vi "Save dat File (Core).vi"(0 "File path in":path, 5 "Attributes":string[][](array[string]), 7 "Channels names":string[](array[string]), 9 "Data":sgl[][](array[numeric]) format="%.2p", 11 "error in":errorcluster, 12 "Cut Data at first NaN":bool=TRUE caption="Cut Data at first NaN? (T)") -> (4 "File path out":path, 15 "error out":errorcluster)   [LabVIEW 2017, in "Nanonis Prog Interface.lvlib"]
doc: "<b>Saves a .dat file.</b>\n\nIt saves the attributes in the header, and then the channels names and the corresponding data into a .dat file.\n\nThis function is the core of the Save dat File function, and it's not password-protected so that the user has access to the code.\n\nIf file dialog and/or automated file naming are needed, the user should use the Save dat File function instead.\n\n<B>File path in</B>: full path input of the saved file.\n<B>Attributes</B>: the first column should be fill in with the attribute name, and the second column with the attribute value.\n<B>Channels names</B>: these are set as column headers in the file. The signals names are available in Signals palette through Signal Names Get function.\n<B>Data</B>: saved data in 2D array format. Each row represents one channel.\n<B>Cut Data at first NaN</B>: optional input to avoid saving Not a Number values into the file. It is set to True by default.\n\n<B>File path out</B>: full path output of the saved fle.\n\n- Nanonis Programming Interface -"
uses:
  Nanonis Prog Interface.lvlib
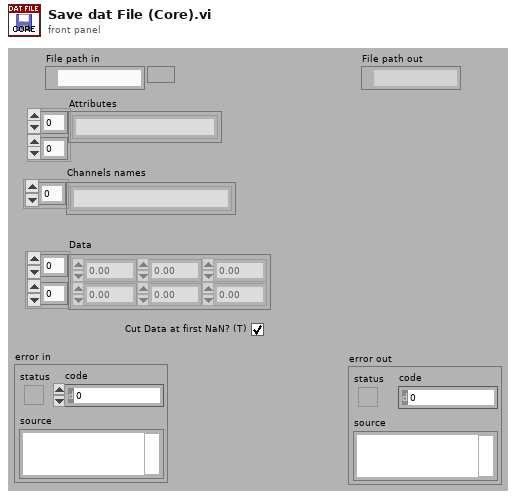
[diagram p1: front panel]
types:
  T1 = enum16{"open", "replace", "create", "open or create", "replace or create", "replace or create with confirmation"}
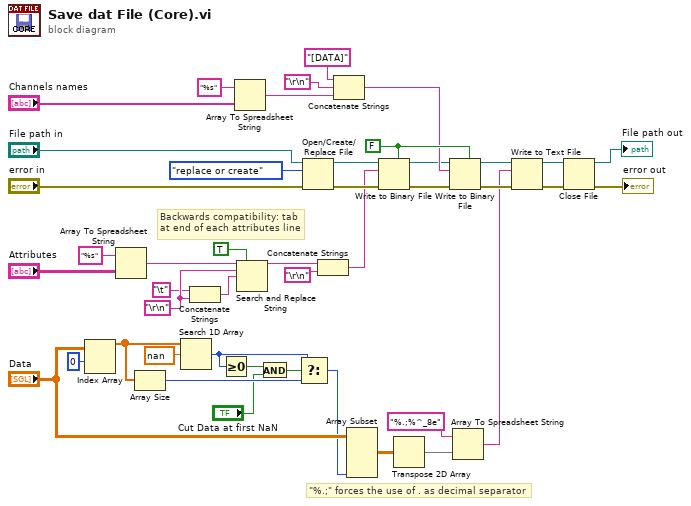
[diagram p0: block diagram]
diagram:
  w4 = "\r\n"
  w33 = FALSE ("prepend array or string size? (T)")
  # "Backwards compatibility: tab at end of each attributes line"
  # "\"%.;\" forces the use of . as decimal separator"
  n1 = Index Array(array="Data", index (row)=0 ("disabled index (col)")) -> (element=w16:sgl[])  [unwired: 1 in]
  n2 = Array To Spreadsheet String(array="Attributes", 3:"%s" ("format string")) -> (spreadsheet string=w6:string)  [unwired: 1 in]
  n3 = Array Size(array=w16) -> (size(s)=w23:i32)
  n4 = Search 1D Array(1D array=w16, element=sgl nan) -> (index of element=w17:i32)  [unwired: 1 in]
  n5 = Concatenate Strings("\t", w4) -> (w2:string)
  n6 = Greater Or Equal To 0?(x=w17) -> (x >= 0?=w20:bool)
  n7 = Array To Spreadsheet String(array="Channels names", 3:"%s" ("format string")) -> (spreadsheet string=w10:string)  [unwired: 1 in]
  n8 = Search and Replace String(replace all?=TRUE ("replace all? (F)"), input string=w6, search string=w4, replace string=w2) -> (result string=w1:string)  [unwired: 4 in, 3 out]
  n9 = And(x=w20, y="Cut Data at first NaN") -> (x .and. y?=w21:bool)
  n10 = Select(t=w17, s=w21, f=w23) -> (s? t:f=w18:i32)
  n11 = Open/Create/Replace File(file path (use dialog)="File path in", error in="error in", operation (0:open)=T1."replace or create") -> (refnum out=w28:refnum<file>, error out=w29:errorcluster)  [unwired: 3 in, 1 out]
  n12 = Concatenate Strings(w1, "\r\n") -> (w12:string)
  n13 = Concatenate Strings("[DATA]" ("new element/subarray"), "\r\n", w10) -> (w32:string)
  n14 = Array Subset(array="Data", length (col)=w18) -> (w34:sgl[][])  [unwired: 3 in]
  n15 = Write to Binary File(file (use dialog)=w28, data=w12, error in=w29, 5:w33) -> (refnum out=w30:refnum<file>, error out=w31:errorcluster)  [unwired: 2 in, 1 out]
  n16 = Transpose 2D Array(2D array=w34) -> (transposed array=w35:sgl[][])
  n17 = Write to Binary File(file (use dialog)=w30, data=w32, error in=w31, 5:w33) -> (refnum out=w37:refnum<file>, error out=w39:errorcluster)  [unwired: 2 in, 1 out]
  n18 = Array To Spreadsheet String(array=w35, 3:"%.;%^_8e" ("format (%.3f)")) -> (spreadsheet string=w38:string)  [unwired: 1 in]
  n19 = Write to Text File(file (use dialog)=w37, text=w38, error in=w39) -> (refnum out=w40:refnum<file>, error out=w41:errorcluster)  [unwired: 1 in, 1 out]
  n20 = Close File(refnum=w40, error in=w41) -> (path=→"File path out":path, error out=→"error out":errorcluster)
